vi "Get all Queue Statuses.vi"(8 "error in (no error)":errorcluster, 9 "Recipes Queue":refnum<queue>, 10 "Saturation Queue":refnum<queue>, 11 "Expansion Queue":refnum<queue>) -> (0 "error out":errorcluster)   [LabVIEW 2017]
uses:
  Expansion/Expansion.lvclass
  Recipes/Recipes.lvclass
  Saturation/Saturation.lvclass
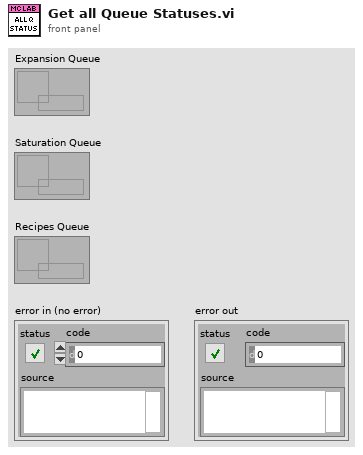
[diagram p1: front panel]
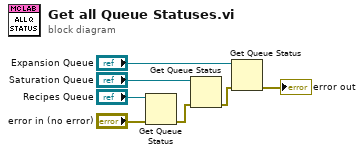
[diagram p0: block diagram]
diagram:
  n1 = Get Queue Status(queue="Recipes Queue", error in (no error)="error in (no error)") -> (error out=w6:errorcluster)  [unwired: 1 in, 7 out]
  n2 = Get Queue Status(queue="Saturation Queue", error in (no error)=w6) -> (error out=w5:errorcluster)  [unwired: 1 in, 7 out]
  n3 = Get Queue Status(queue="Expansion Queue", error in (no error)=w5) -> (error out=→"error out":errorcluster)  [unwired: 1 in, 7 out]
